vi "resetWaveform.vi"(8 "error in (no error)":errorcluster, 11 "Model in":refnum<class "Model.lvclass">) -> (0 "error out":errorcluster, 3 "Model out":refnum<class "Model.lvclass">)   [LabVIEW 2015, in "Model.lvclass"]
uses:
  Model.lvclass
  Model.lvclass/Model.ctl
  WaveformFactory/IWaveformFactory/IWaveformFactory.lvclass
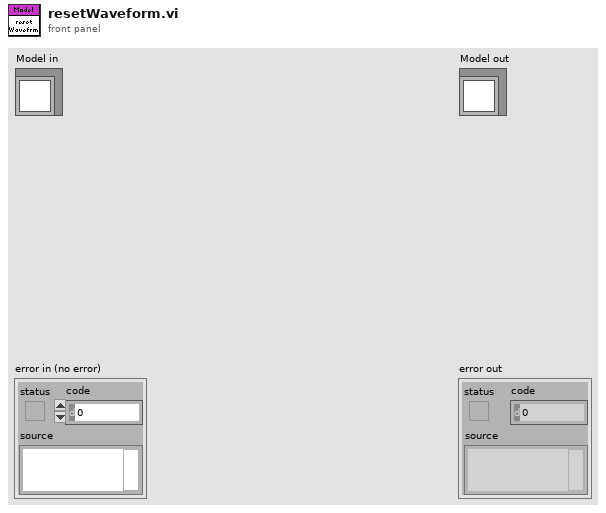
[diagram p1: front panel]
types:
  T1 = typedef "FAMTTypedefs.lvlib/Scan Settings.ctl" = cluster{"Amplitude Scan Settings":T2, "Rate Scan Settings":T3[], "Sample Rate":dbl[unit], "Iterations":dbl, "Amplitude":dbl[unit], "Offset":dbl[unit], "Frequency":dbl[unit], "Waveform":T4, "F1":dbl[unit], "F2":dbl[unit], "Duty Cycle":dbl}
  T2 = typedef "FAMTTypedefs.lvlib/Test Values.ctl" = cluster{"Start Value":dbl, "Stop Value":dbl, "Steps":u16}
  T3 = typedef "ILCCommon.lvlib/ILCConfiguration.lvlib/Scan Rates.ctl" = enum16{"50", "60", "100", "120", "200", "240", "300", "400", "480", "600", "1200", "2400", "4800"}
  T4 = typedef "FAMTTypedefs.lvlib/Waveform.ctl" = enum16{"Sine Wave", "Triangle Wave", "Square Wave", "Sawtooth Wave", "Chirp Wave", "Gaussian Wave"}
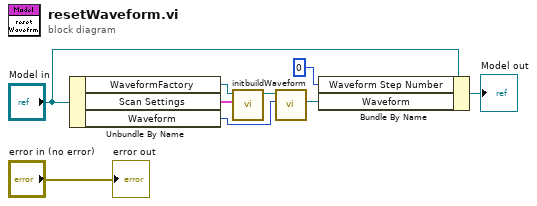
[diagram p0: block diagram]
diagram:
  n1 = Unbundle By Name("Model in") -> ("WaveformFactory"=w5:refnum<class "IWaveformFactory.lvclass">, "Scan Settings"=w6:T1, "Waveform"=w3:T4)
  n2 = call-dynamic "init.vi"("Scan Settings"=w6, "IWaveformFactory in"=w5) -> ("IWaveformFactory out"=w4:refnum<class "IWaveformFactory.lvclass">)  [unwired: 8 in, 1 out]
  n3 = call-dynamic "buildWaveform.vi"("Waveforms"=w3, "IWaveformFactory in"=w4) -> ("Waveform"=w2:refnum<class "IWaveform.lvclass">)  [unwired: 7 in, 2 out]
  n4 = Bundle By Name(cluster="Model in", "Waveform Step Number"=u16 0, "Waveform"=w2) -> (→"Model out":refnum<class "Model.lvclass">)
  "error out" <- "error in (no error)"
